vi "make_color_index_array.vi"(10 "Amplitude Min/Max":T1, 11 "Z array":sgl[](array[numeric])) -> (3 "Color Index Array":i32[](array[numeric]))   [LabVIEW 2020]
uses:
  <vilib>/Native 3D Graph/typedefs/min_max.ctl
  <vilib>/Native 3D Graph/xcontrol/3DPC_SurfacePlot.xctl
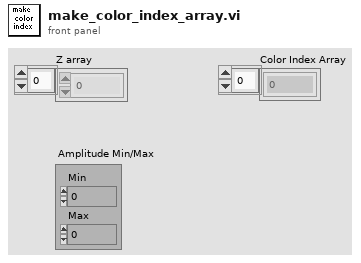
[diagram p1: front panel]
types:
  T1 = typedef "3DPC_SurfacePlot.xctl/min_max.ctl" = cluster{"Min":sgl, "Max":sgl}
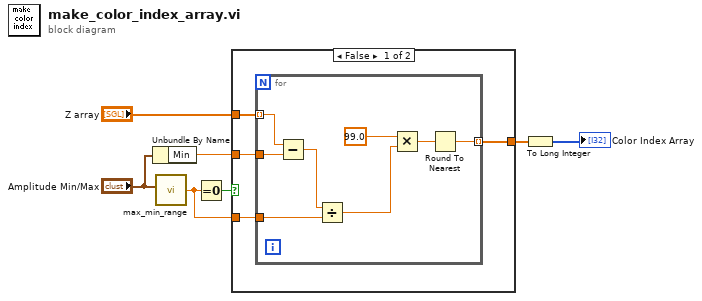
[diagram p0: block diagram]
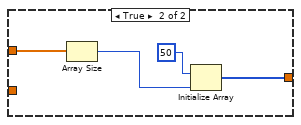
[diagram p2: hidden frame]
diagram:
  n1 = Unbundle By Name("Amplitude Min/Max") -> ("Min"=w5:sgl)
  n2 = call <vilib>:"max_min_range.vi"("Z Min/Max"="Amplitude Min/Max") -> ("Range"=w3:sgl)  [unwired: 8 out]
  n3 = Equal To 0?(x=w3) -> (x = 0?=w4:bool)
  n4 = case shown="False" w4 {
    tunnel: "Z array" -> [w11 w23]
    tunnel: w3 -> [w10 _]
    tunnel: w5 -> [w9 _]
    tunnel: [w8 w20] -> w2
    frame False {
      n5 = for {
        tunnel: w11 -> [w18] mode=indexing
        tunnel: w10 -> [w16]
        tunnel: w9 -> [w17]
        tunnel: [w12] -> w8 mode=indexing
        n6 = Subtract(x=w18, y=w17) -> (x-y=w19:sgl)
        n7 = Divide(x=w19, y=w16) -> (x/y=w15:sgl)
        n8 = Multiply(x=sgl 99.0 ("Number of Colors"), y=w15) -> (x*y=w13:sgl)
        n9 = Round To Nearest(number=w13) -> (nearest integer value=w12:sgl)
      }
    }
    frame True {
      n10 = Array Size(array=w23) -> (size(s)=w22:i32)
      n11 = Initialize Array(50, w22) -> (w20:i32[])
    }
  }
  n12 = To Long Integer(number=w2) -> (32bit integer=→"Color Index Array":i32[])
